vi "Set Cursor to Mouse Click.vi"(8 "Error In":errorcluster, 9 "Vertical":i32, 10 "Horizontal":i32, 11 "RichTextBox Refnum":refnum<k24>) -> (0 "Error Out":errorcluster)   [LabVIEW 2021, in "Notebook.lvlib"]
uses:
  Notebook.lvlib
  System.Windows.Forms
  System.Drawing
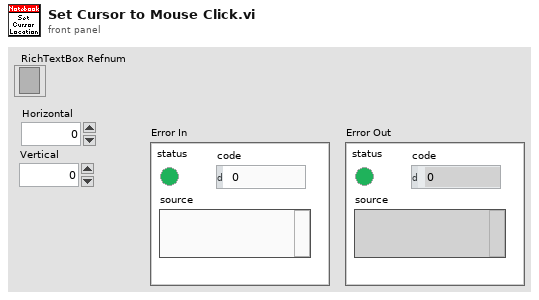
[diagram p1: front panel]
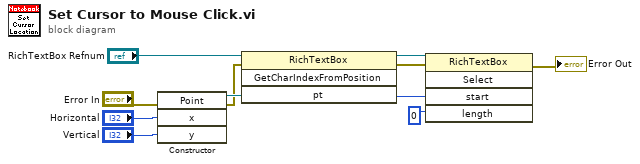
[diagram p0: block diagram]
diagram:
  n1 = constructor class="Point"(error in="Error In", "x"="Horizontal", "y"="Vertical") -> (reference out=w8:refnum<k24>, error out=w3:errorcluster)  [unwired: 2 in, 3 out]
  n2 = invoke class="RichTextBox" method="GetCharIndexFromPosition"(reference="RichTextBox Refnum", error in=w3, "pt"=w8) -> (reference out=w9:refnum<k24>, error out=w2:errorcluster, "GetCharIndexFromPosition"=w11:i32)  [unwired: 1 in, 1 out]
  n3 = invoke class="RichTextBox" method="Select"(reference=w9, error in=w2, "start"=w11, "length"=0) -> (error out=→"Error Out":errorcluster)  [unwired: 1 in, 4 out]
